vi "create_request_builder.vi"(5 "RequestBuilder type":refnum<class "RequestBuilder.lvclass">, 7 "HTTP Method":T1, 8 "error in (no error)":errorcluster, 10 "url":string, 11 "Client in":refnum<class "Client.lvclass">) -> (0 "error out":errorcluster, 2 "RequestBuilder out":refnum<class "RequestBuilder.lvclass">, 3 "Client out":refnum<class "Client.lvclass">)   [LabVIEW 2020, in "reqwest.lvlib" / "Client.lvclass"]
uses:
  Client.lvclass
  RequestBuilder/RequestBuilder.lvclass
  Types/http_method_enum.ctl
  Client.lvclass/Client.ctl
  lv_reqwest_32.dll
  reqwest.lvlib
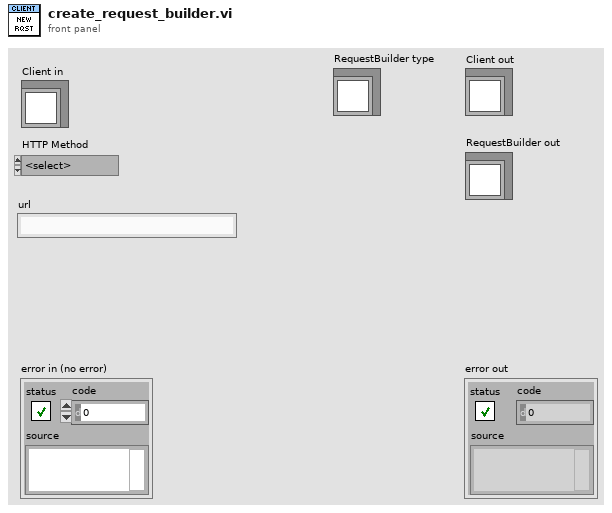
[diagram p1: front panel]
types:
  T1 = typedef "reqwest.lvlib/http_method_enum.ctl" = enum8{"<select>", "GET", "POST", "PUT", "DELETE", "HEAD", "OPTIONS", "CONNECT", "PATCH", "TRACE"}
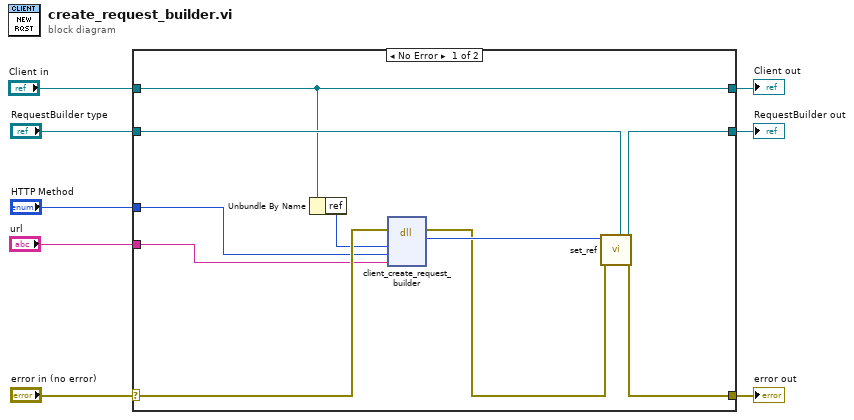
[diagram p0: block diagram]
diagram:
  n1 = case shown="No Error" "error in (no error)" {
    selector: "error in (no error)" -> [w18 w21]
    tunnel: [w10 w21] -> w7
    tunnel: [w14 w20] -> w5
    tunnel: "RequestBuilder type" -> [w13 w20]
    tunnel: "HTTP Method" -> [w17 _]
    tunnel: "url" -> [w16 _]
    tunnel: "Client in" -> [w9 w19]
    tunnel: [w9 w19] -> w1
    frame No Error {
      n2 = Unbundle By Name(w9) -> ("ref"=w12:u64)
      n3 = dll-call lib="C:/Projects/reqwest-rs-labview/lv_src/lv_reqwest_*.*" fn="client_create_request_builder"(error in=w18, "client_ref"=w12, "http_method"=w17, "url"=w16) -> (error out=w11:errorcluster, "request_builder_ref"=w15:u64)  [unwired: 5 in, 1 out]
      n4 = call "set_ref.vi"("ref in"=w13, "error in (no error)"=w11, "ref"=w15) -> ("error out"=w10:errorcluster, "ref out"=w14:refnum<class "RequestBuilder.lvclass">)  [unwired: 7 in]
    }
    frame Error {
    }
  }
  "error out" <- w7
  "RequestBuilder out" <- w5
  "Client out" <- w1
